vi "create.vi"(5 "reporting type":T1, 7 "ID":string, 10 "results reporter":refnum<class "results reporter.lvclass">, 11 "tasks":refnum<class "task.lvclass">[](array[class])) -> (3 "batch task out":refnum<class "batch task.lvclass">)   [LabVIEW 2013, in "batch task.lvclass"]
uses:
  batch task.lvclass
  results reporter/results reporter.lvclass
  reporting type.ctl
  task/task.lvclass
  batch task.lvclass/batch task.ctl
  task/task.lvclass/task.ctl
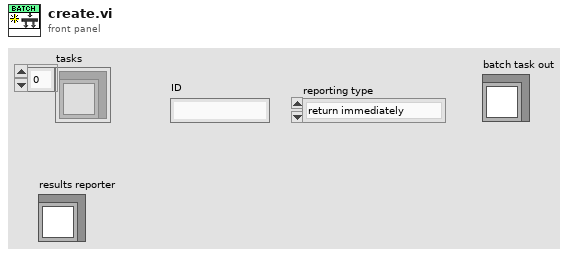
[diagram p1: front panel]
types:
  T1 = typedef "batch task.lvclass/reporting type.ctl" = enum16{"return immediately", "wait on all"}
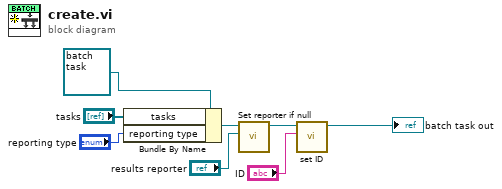
[diagram p0: block diagram]
diagram:
  n1 = Bundle By Name(cluster=refnum<class "batch task.lvclass"> refnum ("batch task in"), "tasks"="tasks", "reporting type"="reporting type") -> (w6:refnum<class "batch task.lvclass">)
  n2 = call "Set reporter if null.vi"("results reporter"="results reporter", "task in"=w6) -> ("task out"=w7:refnum<class "batch task.lvclass">)  [unwired: 9 in]
  n3 = call "set ID.vi"("ID"="ID", "task in"=w7) -> ("task out"=→"batch task out":refnum<class "batch task.lvclass">)  [unwired: 9 in]
